vi "validate against lvparse.vi"() -> ()   [LabVIEW 2014]
uses:
  generate string.vi
  generate false.vi
  generate true.vi
  escape json string.vi
  generate number.vi
  generate array.vi
  generate object.vi
  json generator.lvlib
panel:
  out "cluster same":bool
  out "object string":string
  out "JSON string":string
  out "x != y?":T1
  out "gen error":errorcluster
  out "native err":errorcluster
  out "gen unflat":bool
  out "native unflat":bool
  out "native":dbl
  out "gen":dbl
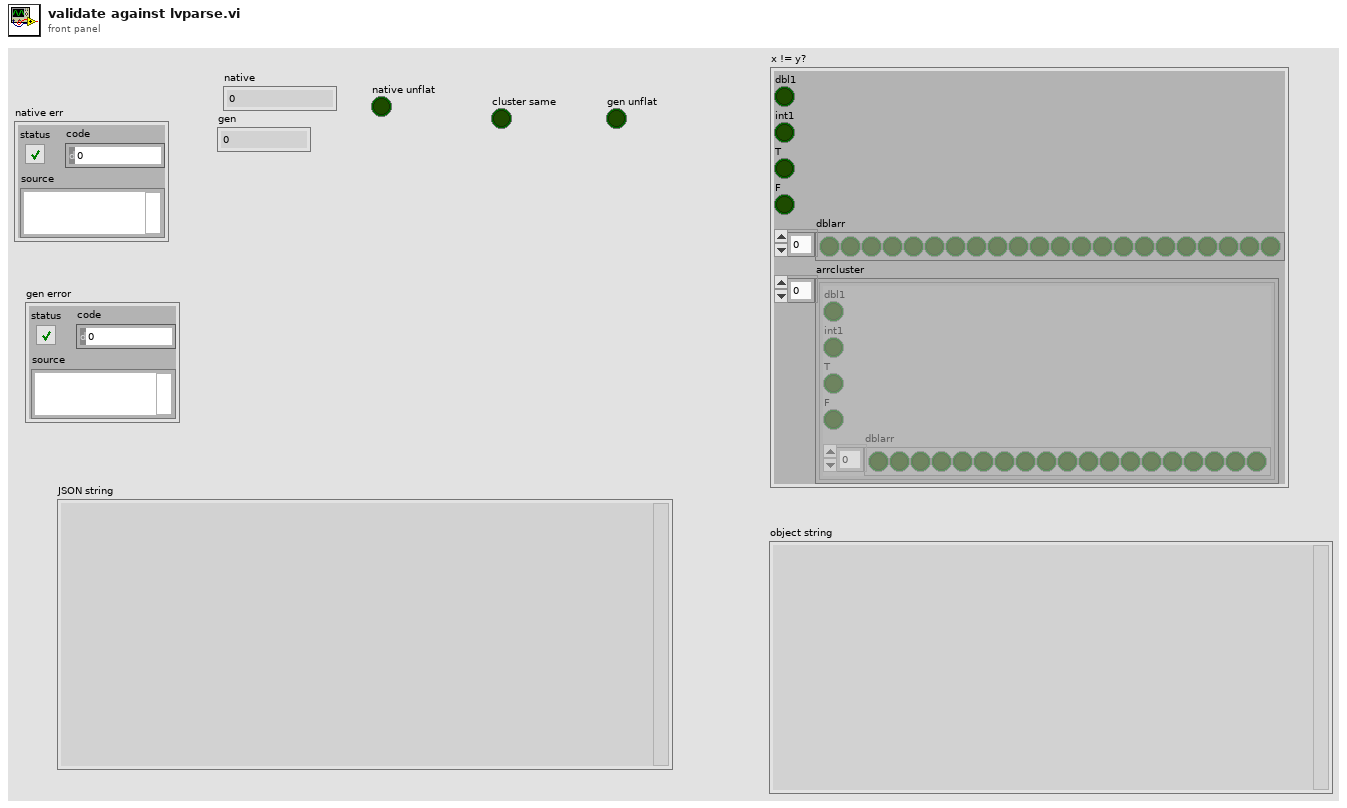
[diagram p1: front panel]
types:
  T1 = cluster{"dbl1":bool, "int1":bool, "T":bool, "F":bool, "dblarr":bool[], "arrcluster":cluster{"dbl1":bool, "int1":bool, "T":bool, "F":bool, "dblarr":bool[]}[]}
  T2 = cluster{"dbl1":dbl, "int1":i32, "T":bool, "F":bool, "dblarr":dbl[], "arrcluster":cluster{"dbl1":dbl, "int1":i32, "T":bool, "F":bool, "dblarr":dbl[]}[]}
  T3 = cluster{"dbl1":dbl, "int1":i32, "T":bool, "F":bool, "dblarr":dbl[]}
  T4 = cluster{"dbl1":dbl, "int1":i32, "T":bool, "F":bool, "dblarr":dbl[]}[]
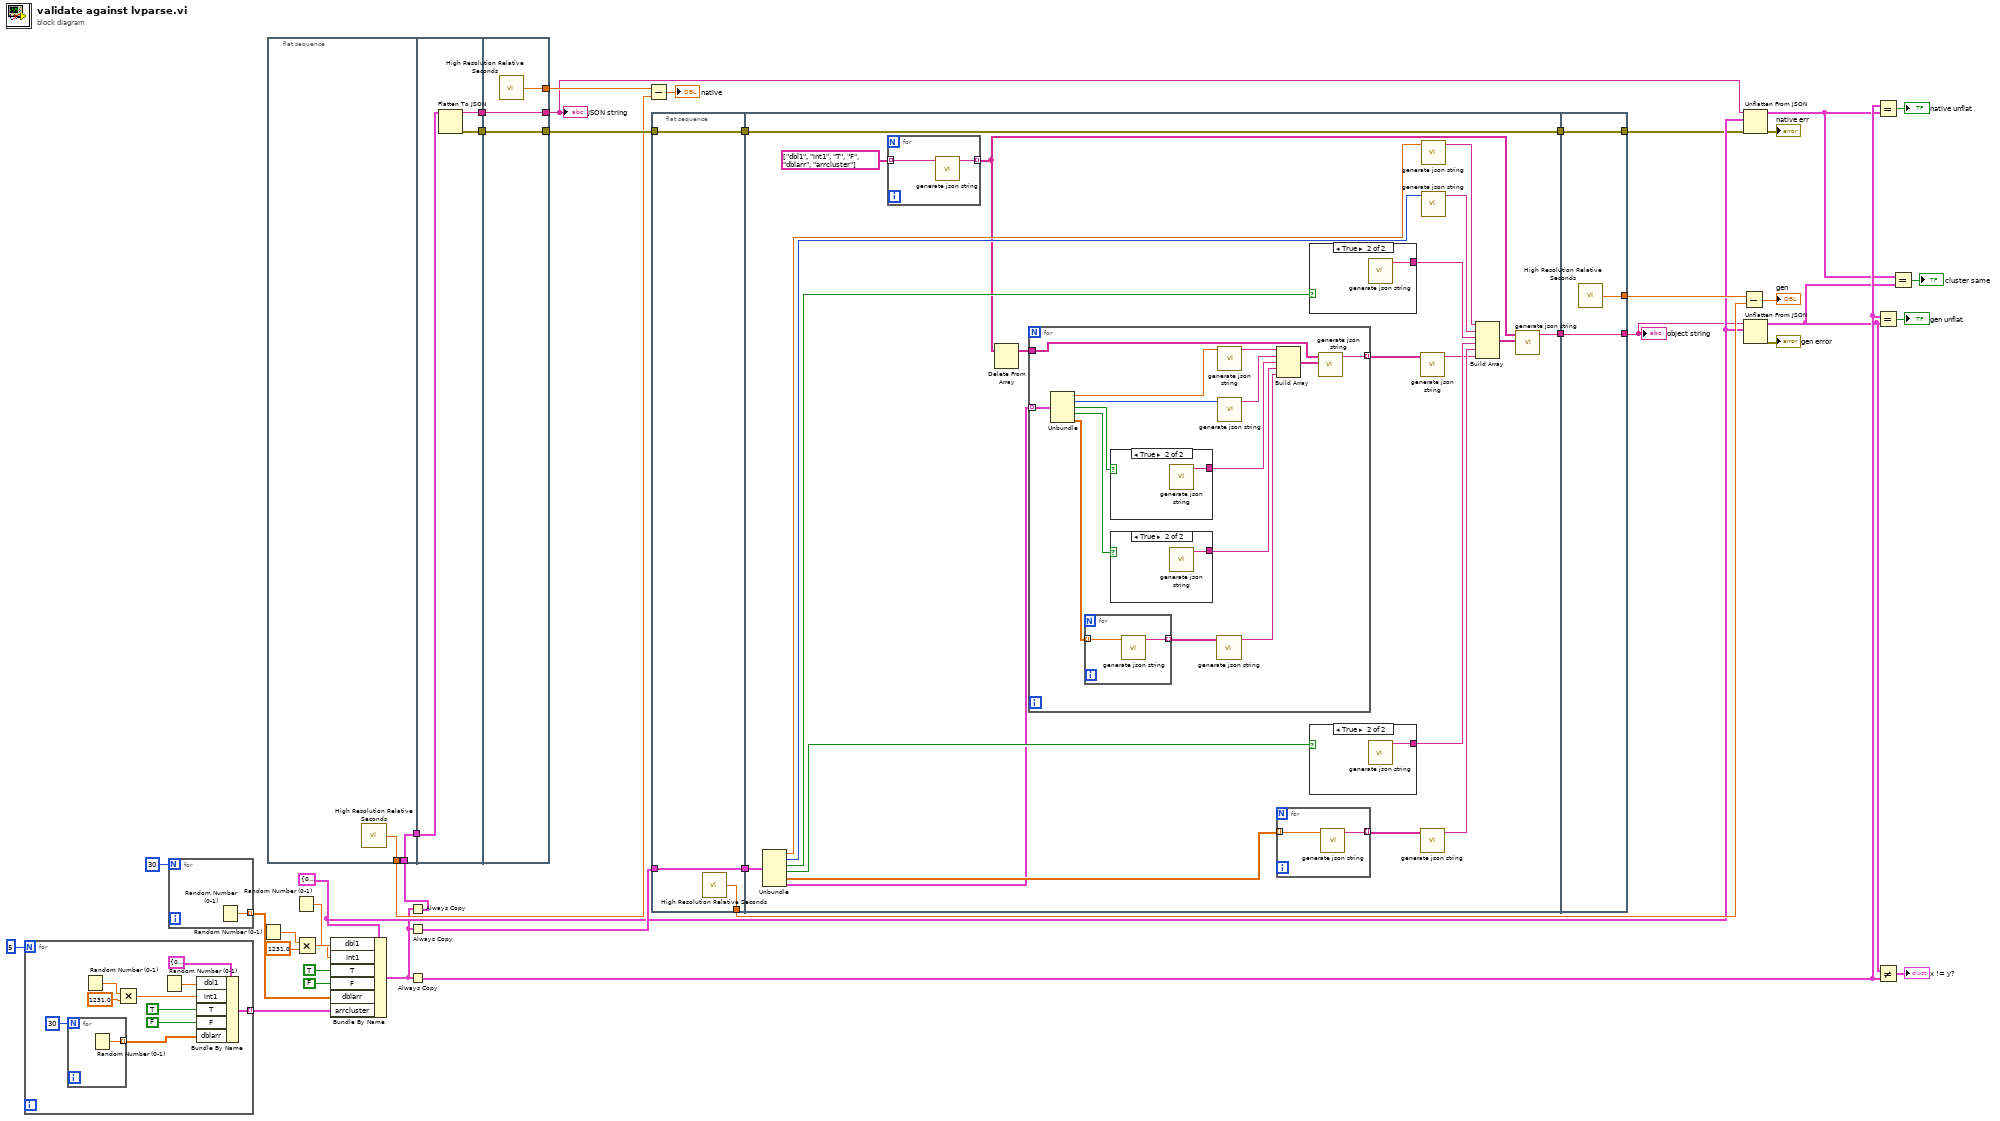
[diagram p0: block diagram]
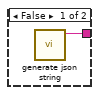
[diagram p2: hidden frame]
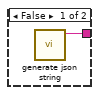
[diagram p3: hidden frame]
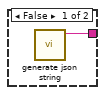
[diagram p4: hidden frame]
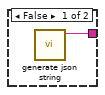
[diagram p5: hidden frame]
diagram:
  w21 = T2 {"dbl1"=0.0, "int1"=0, "T"=TRUE, "F"=FALSE, "dblarr"=[], "arrcluster"=[]}
  n1 = for {
    N: 5 -> [_]
    tunnel: [w49] -> w14 mode=indexing
    n2 = for {
      N: 30 -> [_]
      tunnel: [w51] -> w47 mode=indexing
      n3 = Random Number (0-1)() -> (number: 0 to 1=w51:dbl)
    }
    n4 = Random Number (0-1)() -> (number: 0 to 1=w43:dbl)
    n5 = Multiply(x=w43, y=1231.0) -> (x*y=w42:dbl)
    n6 = Random Number (0-1)() -> (number: 0 to 1=w41:dbl)
    n7 = Bundle By Name(cluster=T3 {"dbl1"=0.0, "int1"=0, "T"=TRUE, "F"=FALSE, "dblarr"=[]}, "dbl1"=w41, "int1"=w42, "T"=TRUE, "F"=FALSE, "dblarr"=w47) -> (w49:T3)
  }
  n8 = for {
    N: 30 -> [_]
    tunnel: [w52] -> w30 mode=indexing
    n9 = Random Number (0-1)() -> (number: 0 to 1=w52:dbl)
  }
  n10 = Random Number (0-1)() -> (number: 0 to 1=w34:dbl)
  n11 = flat-sequence {
    tunnel: [w54] -> w22
    tunnel: [w53] -> w3
    tunnel: w2 -> [w53]
    tunnel: [w57] -> w26
    tunnel: [w56] -> w25
    tunnel: w3 -> [w55]
    tunnel: [w59] -> w20
    tunnel: [w60] -> w29
    tunnel: w26 -> [w60]
    tunnel: w25 -> [w59]
    tunnel: [w58] -> w23
    frame #0 {
      n12 = call <vilib>:"High Resolution Relative Seconds.vi"() -> ("relative seconds"=w54:dbl)
    }
    frame #1 {
      n13 = Flatten To JSON(anything=w55) -> (JSON string=w56:string, 11:w57:errorcluster)  [unwired: 2 in]
    }
    frame #2 {
      n14 = call <vilib>:"High Resolution Relative Seconds.vi"() -> ("relative seconds"=w58:dbl)
    }
  }
  n15 = Random Number (0-1)() -> (number: 0 to 1=w35:dbl)
  n16 = Multiply(x=w34, y=1231.0) -> (x*y=w32:dbl)
  n17 = Bundle By Name(cluster=w21, "dbl1"=w35, "int1"=w32, "T"=TRUE, "F"=FALSE, "dblarr"=w30, "arrcluster"=w14) -> (w17:T2)
  n18 = Always Copy(1:w17) -> (0:w2:T2)
  n19 = Always Copy(1:w17) -> (0:w27:T2)
  n20 = Always Copy(1:w17) -> (0:w7:T2)
  n21 = Subtract(x=w23, y=w22) -> (x-y=→"native":dbl)
  n22 = flat-sequence {
    tunnel: [w63] -> w39
    tunnel: w29 -> [w61]
    tunnel: [w62] -> w28
    tunnel: w27 -> [w62]
    tunnel: [w61] -> w8
    tunnel: w28 -> [w84]
    tunnel: [w83] -> w12
    tunnel: [w67] -> w9
    tunnel: w8 -> [w67]
    tunnel: [w116] -> w40
    tunnel: [w115] -> w11
    tunnel: w12 -> [w115]
    tunnel: [w114] -> w10
    tunnel: w9 -> [w114]
    frame #0 {
      n23 = call <vilib>:"High Resolution Relative Seconds.vi"() -> ("relative seconds"=w63:dbl)
    }
    frame #1 {
      n24 = Unbundle(w84) -> ("dbl1"=w80:dbl, "int1"=w81:i32, "T"=w82:bool, "F"=w74:bool, "dblarr"=w71:dbl[], "arrcluster"=w69:T4)
      n25 = for {
        tunnel: string[] ["dbl1", "int1", "T", "F", "dblarr", "arrcluster"] ("json string keys") -> [w86] mode=indexing
        tunnel: [w85] -> w65 mode=indexing
        n26 = call-poly "generate json string.vi"("base string"=w86) -> ("json string"=w85:string)  [unwired: 10 in]
      }
      n27 = Delete From Array(array=w65) -> (array with subset deleted=w64:string[])  [unwired: 2 in, 1 out]
      n28 = for {
        tunnel: w69 -> [w101] mode=indexing
        tunnel: [w100] -> w68 mode=indexing
        tunnel: w64 -> [w87]
        n29 = Unbundle(w101) -> ("dbl1"=w92:dbl, "int1"=w91:i32, "T"=w90:bool, "F"=w88:bool, "dblarr"=w89:dbl[])
        n30 = for {
          tunnel: w89 -> [w103] mode=indexing
          tunnel: [w102] -> w99 mode=indexing
          n31 = call-poly "generate json string.vi"("number"=w103) -> ("nunber string"=w102:string)  [unwired: 10 in]
        }
        n32 = case shown="True" w90 {
          tunnel: [w106 w107] -> w94
          frame False {
            n33 = call-poly "generate json string.vi"() -> ("json string"=w106:string)  [unwired: 11 in]
          }
          frame True {
            n34 = call-poly "generate json string.vi"() -> ("json string"=w107:string)  [unwired: 11 in]
          }
        }
        n35 = case shown="True" w88 {
          tunnel: [w104 w105] -> w93
          frame False {
            n36 = call-poly "generate json string.vi"() -> ("json string"=w104:string)  [unwired: 11 in]
          }
          frame True {
            n37 = call-poly "generate json string.vi"() -> ("json string"=w105:string)  [unwired: 11 in]
          }
        }
        n38 = call-poly "generate json string.vi"("json strings"=w99) -> ("array string"=w98:string)  [unwired: 10 in]
        n39 = call-poly "generate json string.vi"("number"=w92) -> ("nunber string"=w96:string)  [unwired: 10 in]
        n40 = call-poly "generate json string.vi"("number"=w91) -> ("nunber string"=w95:string)  [unwired: 10 in]
        n41 = Build Array(w96, w95, w94, w93, w98) -> (w97:string[])
        n42 = call-poly "generate json string.vi"("json string values"=w97, "json string keys"=w87) -> ("object string"=w100:string)  [unwired: 9 in]
      }
      n43 = for {
        tunnel: w71 -> [w109] mode=indexing
        tunnel: [w108] -> w70 mode=indexing
        n44 = call-poly "generate json string.vi"("number"=w109) -> ("nunber string"=w108:string)  [unwired: 10 in]
      }
      n45 = case shown="True" w82 {
        tunnel: [w112 w113] -> w76
        frame False {
          n46 = call-poly "generate json string.vi"() -> ("json string"=w112:string)  [unwired: 11 in]
        }
        frame True {
          n47 = call-poly "generate json string.vi"() -> ("json string"=w113:string)  [unwired: 11 in]
        }
      }
      n48 = case shown="True" w74 {
        tunnel: [w110 w111] -> w75
        frame False {
          n49 = call-poly "generate json string.vi"() -> ("json string"=w110:string)  [unwired: 11 in]
        }
        frame True {
          n50 = call-poly "generate json string.vi"() -> ("json string"=w111:string)  [unwired: 11 in]
        }
      }
      n51 = call-poly "generate json string.vi"("json strings"=w68) -> ("array string"=w72:string)  [unwired: 10 in]
      n52 = call-poly "generate json string.vi"("json strings"=w70) -> ("array string"=w73:string)  [unwired: 10 in]
      n53 = call-poly "generate json string.vi"("number"=w80) -> ("nunber string"=w79:string)  [unwired: 10 in]
      n54 = call-poly "generate json string.vi"("number"=w81) -> ("nunber string"=w78:string)  [unwired: 10 in]
      n55 = Build Array(w79, w78, w76, w75, w73, w72) -> (w77:string[])
      n56 = call-poly "generate json string.vi"("json string values"=w77, "json string keys"=w65) -> ("object string"=w83:string)  [unwired: 9 in]
    }
    frame #2 {
      n57 = call <vilib>:"High Resolution Relative Seconds.vi"() -> ("relative seconds"=w116:dbl)
    }
  }
  n58 = Subtract(x=w40, y=w39) -> (x-y=→"gen":dbl)
  n59 = Unflatten From JSON(JSON string=w20, type and defaults=w21, error in (no error)=w10) -> (value=w5:T2, error out=→"native err":errorcluster)  [unwired: 4 in]
  n60 = Unflatten From JSON(JSON string=w11, type and defaults=w21) -> (value=w4:T2, error out=→"gen error":errorcluster)  [unwired: 5 in]
  n61 = Equal?(x=w7, y=w5) -> (x = y?=→"native unflat":bool)
  n62 = Equal?(x=w7, y=w4) -> (x = y?=→"gen unflat":bool)
  n63 = Not Equal?(x=w4, y=w7) -> (x != y?=→"x != y?":T1)
  n64 = Equal?(x=w5, y=w4) -> (x = y?=→"cluster same":bool)
  "JSON string" <- w20
  "object string" <- w11
